vi "sCMOS_init_TL.vi"(3 "error in":errorcluster, 4 "Start acquisition":bool, 5 "handle":u32) -> (0 "error out":errorcluster {"code" format="%.0x"})   [LabVIEW 2015]
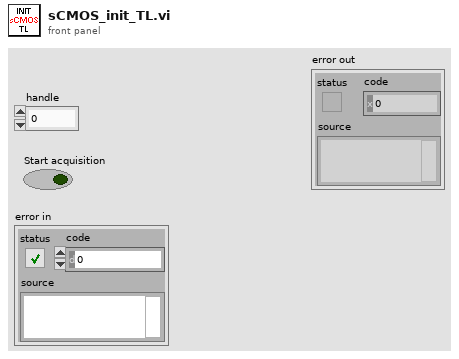
[diagram p1: front panel]
types:
  T1 = cluster{"Mode":u32, "Polarity":u32, "Times":u32, "Delay":dbl}
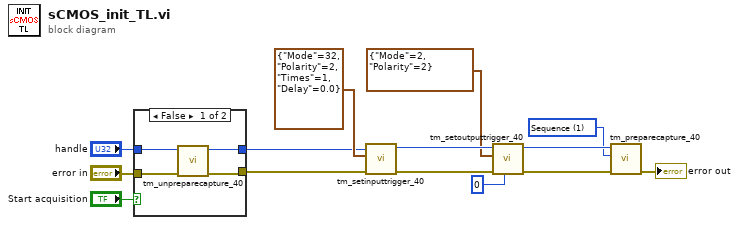
[diagram p0: block diagram]
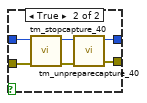
[diagram p2: hidden frame]
diagram:
  w2 = 1 items=["Snap", "Sequence"] ("Capture mode")
  n1 = case shown="False" "Start acquisition" {
    tunnel: "error in" -> [w17 w24]
    tunnel: [w16 w20] -> w5
    tunnel: "handle" -> [w18 w23]
    tunnel: [w15 w19] -> w6
    frame False {
      n2 = call <userlib>:"tm_unpreparecapture_40.vi"("error in (no error)"=w17, "Handle in"=w18) -> ("error out"=w16:errorcluster, "Handle out"=w15:u32)  [unwired: 8 in]
    }
    frame True {
      n3 = call <userlib>:"tm_stopcapture_40.vi"("error in (no error)"=w24, "Handle in"=w23) -> ("error out"=w22:errorcluster, "Handle out"=w21:u32)  [unwired: 8 in]
      n4 = call <userlib>:"tm_unpreparecapture_40.vi"("error in (no error)"=w22, "Handle in"=w21) -> ("error out"=w20:errorcluster, "Handle out"=w19:u32)  [unwired: 8 in]
    }
  }
  n5 = call <userlib>:"tm_setinputtrigger_40.vi"("error in (no error)"=w5, "Parameters"=T1 {"Mode"=32, "Polarity"=2, "Times"=1, "Delay"=0.0}, "Handle in"=w6) -> ("error out"=w11:errorcluster, "Handle out"=w10:u32)  [unwired: 7 in]
  n6 = call <userlib>:"tm_setoutputtrigger_40.vi"("Port"=0, "error in (no error)"=w11, "Type"=cluster{"Mode":u32, "Polarity":u32} {"Mode"=2, "Polarity"=2}, "Handle in"=w10) -> ("error out"=w3:errorcluster, "Handle out"=w4:u32)  [unwired: 6 in]
  n7 = call <userlib>:"tm_preparecapture_40.vi"("error in (no error)"=w3, "Capture mode"=w2, "Handle in"=w4) -> ("error out"=→"error out":errorcluster)  [unwired: 5 in, 3 out]
